vi "Randomized Start Positions.vi"(10 "Player Count":i32, 11 "Size":i32) -> (3 "Positions[]":T1[](array[typedef]))   [LabVIEW 2020, in "SquareBattle.lvlib" / "Game.lvclass"]
uses:
  Game.lvclass
  Position.ctl
  SquareBattle.lvlib
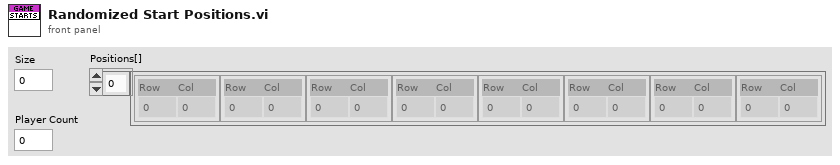
[diagram p1: front panel]
types:
  T1 = typedef "SquareBattle.lvlib/Position.ctl" = cluster{"Row":i32, "Col":i32}
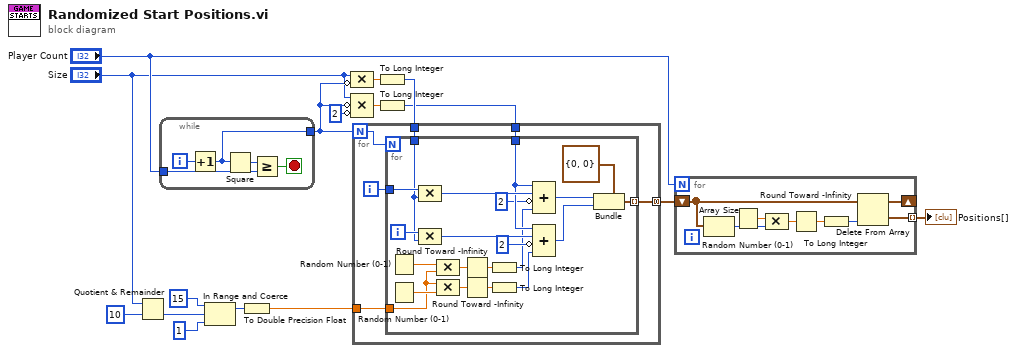
[diagram p0: block diagram]
diagram:
  n1 = Quotient & Remainder(x="Size", y=10) -> (floor(x/y)=w5:i32)  [unwired: 1 out]
  n2 = while {
    tunnel: "Player Count" -> [w19]
    tunnel: [w18] -> w14
    i -> [w21]
    stop <- w20 stop-if-true
    n3 = Increment(x=w21) -> (x+1=w18:i32)
    n4 = Square(x=w18) -> (x^2=w17:i32)
    n5 = Greater Or Equal?(x=w17, y=w19) -> (x >= y?=w20:bool)
  }
  n6 = In Range and Coerce(upper limit=15, x=w5, lower limit=1) -> (coerced(x)=w2:i32)  [unwired: 1 out]
  n7 = To Double Precision Float(number=w2) -> (double precision float=w1:dbl)
  n8 = Compound Arithmetic op=MULTIPLY("Size", invert w14) -> (w16:dbl)
  n9 = Compound Arithmetic op=MULTIPLY("Size", invert w14, invert 2 ("value")) -> (w15:dbl)
  n10 = To Long Integer(number=w16) -> (32bit integer=w12:i32)
  n11 = To Long Integer(number=w15) -> (32bit integer=w11:i32)
  n12 = for {
    N: w14 -> [w27]
    tunnel: w12 -> [w25]
    tunnel: w11 -> [w24]
    tunnel: [w23] -> w9 mode=concatenating
    tunnel: w1 -> [w22]
    i -> [w26]
    n13 = for {
      N: w27 -> [_]
      tunnel: w26 -> [w48]
      tunnel: w25 -> [w46]
      tunnel: w24 -> [w43]
      tunnel: [w40] -> w23 mode=indexing
      tunnel: w22 -> [w28]
      i -> [w47]
      n14 = Random Number (0-1)() -> (number: 0 to 1=w37:dbl)
      n15 = Random Number (0-1)() -> (number: 0 to 1=w36:dbl)
      n16 = Compound Arithmetic op=MULTIPLY(w48, w46) -> (w45:i32)
      n17 = Compound Arithmetic op=MULTIPLY(w47, w46) -> (w44:i32)
      n18 = Compound Arithmetic op=MULTIPLY(w37, w28) -> (w35:dbl)
      n19 = Compound Arithmetic op=MULTIPLY(w28, w36) -> (w34:dbl)
      n20 = Round Toward -Infinity(1:w35) -> (0:w33:dbl)
      n21 = Round Toward -Infinity(1:w34) -> (0:w31:dbl)
      n22 = To Long Integer(number=w33) -> (32bit integer=w32:i32)
      n23 = To Long Integer(number=w31) -> (32bit integer=w30:i32)
      n24 = Compound Arithmetic op=ADD(w43, w45, invert 2 ("value"), w32) -> (w42:i32)
      n25 = Compound Arithmetic op=ADD(w43, w44, invert 2 ("value"), w30) -> (w41:i32)
      n26 = Bundle(cluster=T1 {"Row"=0, "Col"=0} ("Position"), "Row"=w42, "Col"=w41) -> (w40:T1)
    }
  }
  n27 = for {
    N: "Player Count" -> [_]
    shift-right: [w50] -> _
    shift-left: w9 -> [w52]
    tunnel: [w49] -> w8 mode=indexing
    n28 = Array Size(array=w52) -> (size(s)=w53:i32)
    n29 = Random Number (0-1)() -> (number: 0 to 1=w54:dbl)
    n30 = Compound Arithmetic op=MULTIPLY(w54, w53) -> (w55:dbl)
    n31 = Round Toward -Infinity(1:w55) -> (0:w56:dbl)
    n32 = To Long Integer(number=w56) -> (32bit integer=w51:i32)
    n33 = Delete From Array(array=w52, index=w51) -> (deleted portion=w49:T1, array with subset deleted=w50:T1[])  [unwired: 1 in]
  }
  "Positions[]" <- w8
